vi "Get List of Synced Monkeys.vi"(8 "error in (no error)":errorcluster, 11 "Tamer in":refnum<class "Tamer.lvclass">) -> (0 "error out":errorcluster, 2 "Synced Monkeys":string[](array[string]), 3 "Tamer out":refnum<class "Tamer.lvclass">)   [LabVIEW 2020, in "CIRCUS_uServices.lvlib" / "Tamer.lvlib" / "Tamer.lvclass"]
uses:
  Tamer.lvclass
  Tamer.lvclass/Tamer.ctl
  TALOS/TALOS_PPL.lvlibp
  C:/Users/marco/Documents/GitHub_Lab/CIRCUS/TALOS/TALOS_PPL.lvlibp/Father of all uServices/Father of all uServices/Father of all uServices.lvclass
  C:/Users/marco/Documents/GitHub_Lab/CIRCUS/TALOS/TALOS_PPL.lvlibp/Ancestor/Ancestor/Ancestor.lvclass
  C:/Users/marco/Documents/GitHub_Lab/CIRCUS/TALOS/Actor Framework.lvlibp/1abvi3w/vi.lib/ActorFramework/Actor/Actor.lvclass
  C:/Users/marco/Documents/GitHub_Lab/CIRCUS/CIRCUS uServices et al/Tamer/Tamer.lvclass
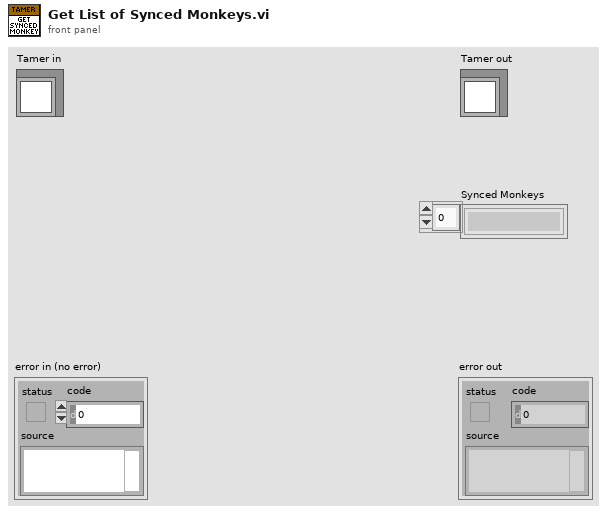
[diagram p1: front panel]
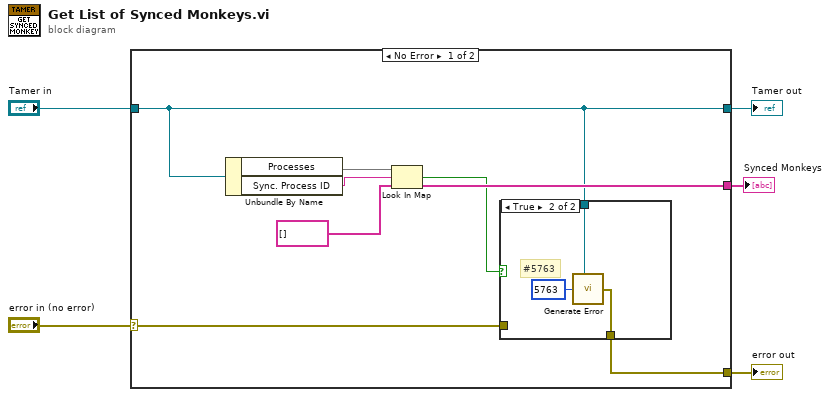
[diagram p0: block diagram]
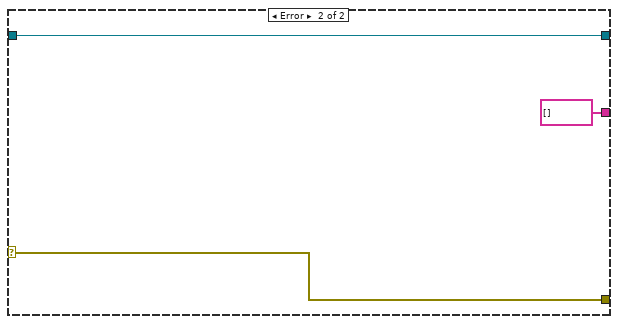
[diagram p3: hidden frame]
diagram:
  n1 = case shown="No Error" "error in (no error)" {
    selector: "error in (no error)" -> [w6 w20]
    tunnel: [w7 w20] -> w4
    tunnel: [w8 w19] -> w2
    tunnel: "Tamer in" -> [w8 w19]
    tunnel: [w11 string[] [] ("Monkeys")] -> w1
    frame No Error {
      n2 = Unbundle By Name(w8) -> ("Processes"=w13:map{string, string[]}, "Sync. Process ID"=w12:string)
      n3 = Look In Map(map=w13, key=w12, default value=string[] []) -> (key not found?=w9:bool, value=w11:string[])
      n4 = case shown="True" w9 {
        tunnel: w8 -> [_ w17]
        tunnel: [w14 w16] -> w7
        tunnel: w6 -> [w14 _]
        frame False {
        }
        frame True {
          # "#5763"
          n5 = call "Generate Error.vi"("Class"=w17, "Error Code"=5763) -> ("error out"=w16:errorcluster)  [unwired: 5 in]
        }
      }
    }
    frame Error {
    }
  }
  "error out" <- w4
  "Tamer out" <- w2
  "Synced Monkeys" <- w1
